vi "CreateWriterFromLib.vi"(0 "LibPath/LvLibRef":variant, 5 "error in":errorcluster) -> (14 "LibWriter":refnum<class "LibWriter.lvclass">, 15 "LvLibRef":refnum<vi>, 19 "error out":errorcluster)   [LabVIEW 2014, in "LibWriter.lvclass"]
uses:
  <resource>/Framework/Providers/Open_GDS/ClassProviders/LibProvider_BaseClassInterface/LibWriter_class/ClassWriter_class/LibWriter.lvclass
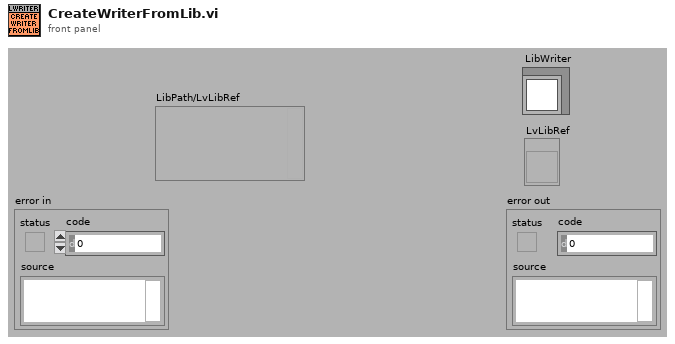
[diagram p1: front panel]
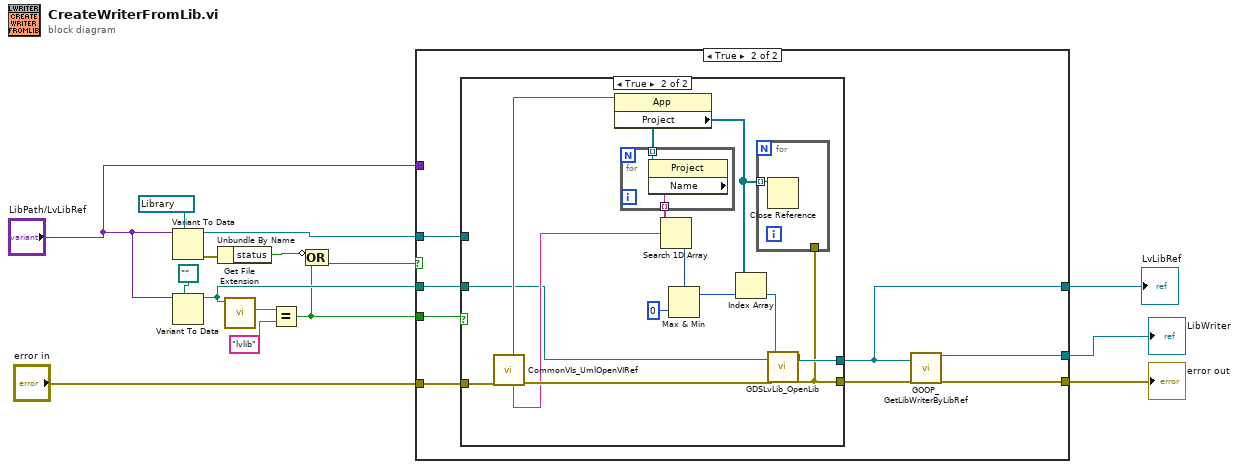
[diagram p0: block diagram]
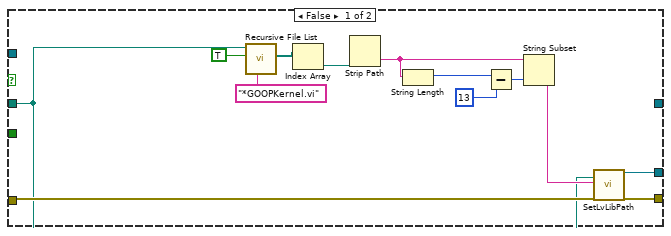
[diagram p2: hidden frame]
diagram:
  n1 = Variant To Data(type=refnum<vi> refnum ("LVClass.Open"), Variant="LibPath/LvLibRef") -> (data=w1:refnum<vi>, error out=w7:errorcluster)  [unwired: 1 in]
  n2 = Variant To Data(type=path "", Variant="LibPath/LvLibRef") -> (data=w3:path)  [unwired: 1 in, 1 out]
  n3 = Unbundle By Name(w7) -> ("status"=w6:bool)
  n4 = call <vilib>:"Get File Extension.vi"("file"=w3) -> ("lowercase file extension"=w9:string)  [unwired: 7 in, 3 out]
  n5 = Equal?(x=w9, y="lvlib") -> (x = y?=w2:bool)
  n6 = Compound Arithmetic op=OR(invert w6, w2) -> (w4:bool)
  n7 = case shown="True" w4 {
    tunnel: "error in" -> [w21 w35]
    tunnel: [w19 w34] -> w14
    tunnel: [w18 w33] -> w13
    tunnel: "LibPath/LvLibRef" -> [_ _]
    tunnel: [_ w32] -> w12
    tunnel: w3 -> [w17 w31]
    tunnel: w2 -> [_ w30]
    tunnel: w1 -> [_ w29]
    frame False {
      n8 = call <vilib>:"Recursive File List.vi"("pattern"="*GOOPKernel.vi", "Treat LLBs as Folders?"=TRUE, "Folder Path"=w17) -> ("All Files in Dir"=w23:path[])  [unwired: 4 in, 4 out]
      n9 = Index Array(array=w23) -> (element=w22:path)  [unwired: 1 in]
      n10 = Strip Path(path=w22) -> (name=w27:string)  [unwired: 1 out]
      n11 = String Length(string=w27) -> (length=w26:i32)
      n12 = Subtract(x=w26, y=13) -> (x-y=w25:i32)
      n13 = String Subset(string=w27, length (rest)=w25) -> (substring=w20:string)  [unwired: 1 in]
      n14 = call <resource>:"SetLvLibPath.vi"("LibPath"=w17, "LibName"=w20, "error in (no error)"=w21) -> ("LibWriter"=w19:refnum<class "LibWriter.lvclass">, "error out"=w18:errorcluster)  [unwired: 15 in]
    }
    frame True {
      n15 = case shown="True" w30 {
        tunnel: w35 -> [w36 w50]
        tunnel: [w36 w38] -> w33
        tunnel: [w37 w41] -> w32
        tunnel: w31 -> [_ w40]
        tunnel: w29 -> [w37 _]
        frame False {
        }
        frame True {
          n16 = call <resource>:"CommonVIs_UmlOpenVIRef.vi"("error in"=w50) -> ("error out"=w49:errorcluster, "ProjectNameOut"=w43:string, "AppRefOut"=w44:refnum<vi>)  [unwired: 7 in, 1 out]
          n17 = property class="App"(reference=w44) -> ("Project"=w39:refnum<vi>[])  [unwired: 1 in, 2 out]
          n18 = for {
            tunnel: w39 -> [w53] mode=indexing
            tunnel: [w52] -> w48 mode=indexing
            n19 = property class="Project"(reference=w53) -> ("Name"=w52:string)  [unwired: 1 in, 2 out]
          }
          n20 = Search 1D Array(1D array=w48, element=w43) -> (index of element=w47:i32)  [unwired: 1 in]
          n21 = Max & Min(x=w47, y=0) -> (max(x,y)=w45:i32)  [unwired: 1 out]
          n22 = Index Array(array=w39, index=w45) -> (element=w42:refnum<vi>)
          n23 = call <resource>:"GDSLvLib_OpenLib.vi"("LibToOpen"=w40, "error in (no error)"=w49, "Project/ApplicationRef(If empty, currect active project will be used)"=w42) -> ("LvLib"=w41:refnum<vi>, "error out"=w38:errorcluster)  [unwired: 15 in]
          n24 = for {
            tunnel: w39 -> [w51] mode=indexing
            tunnel: w38 -> [_]
            n25 = Close Reference(reference=w51) -> ()  [unwired: 1 in, 1 out]
          }
        }
      }
      n26 = call <resource>:"GOOP_GetLibWriterByLibRef.vi"("Library Refnum"=w32, "error in (no error)"=w33) -> ("LibWriter"=w34:refnum<class "LibWriter.lvclass">)  [unwired: 16 in, 1 out]
    }
  }
  "LibWriter" <- w14
  "error out" <- w13
  "LvLibRef" <- w12
